vi "MT Decimate Oversampled Waveform.vi"(0 "input complex waveform":T1={"t0"=0.0, "dt"=1.0, "Y"=[]} {"Y" format="%.3f"; "dt" format="%^.2e"; "t0" format="%.4f"}, 5 "decimation factor":i32=16, 7 "offset":i32, 11 "error in (no error)":errorcluster, 13 "reset? (T)":bool=TRUE) -> (4 "output complex waveform":T1 {"Y" format="%.3f"; "dt" format="%^.2e"; "t0" format="%.4f"}, 15 "error out":errorcluster)   [LabVIEW 2020, in "niDMT.lvlib"]
doc: "Decimates the <B>input complex waveform</B> and returns the decimated <B>output complex waveform</B>. Use this VI to decimate the matched filtered waveform at the output of the MT Matched Filter VI to recover the symbols corresponding to the ideal symbol timing location."
uses:
  <vilib>/addons/Modulation/niDMT.lvlib
  <vilib>/addons/Modulation/Analog/controls/Complex Data Waveform.ctl
  <vilib>/addons/Modulation/Analog/support/Validators/mod_Validate Complex Waveform.vi
  <vilib>/addons/Modulation/Analog/support/Validators/mod_WFErrorHandler.vi
  <vilib>/addons/Modulation/niAMT.lvlib
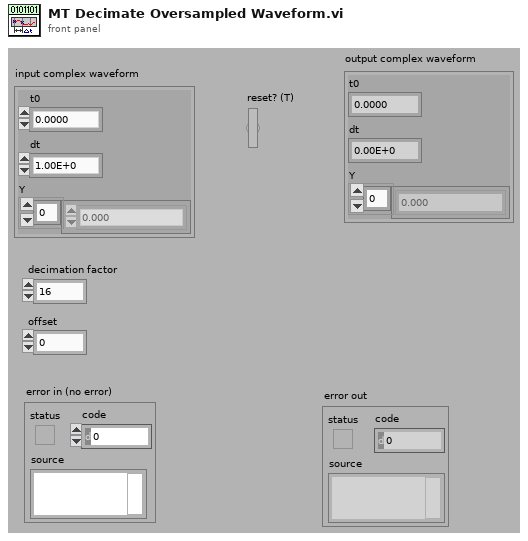
[diagram p1: front panel]
types:
  T1 = typedef "niAMT.lvlib/Complex Data Waveform.ctl" = cluster{"t0":dbl, "dt":dbl, "Y":cdb[]}
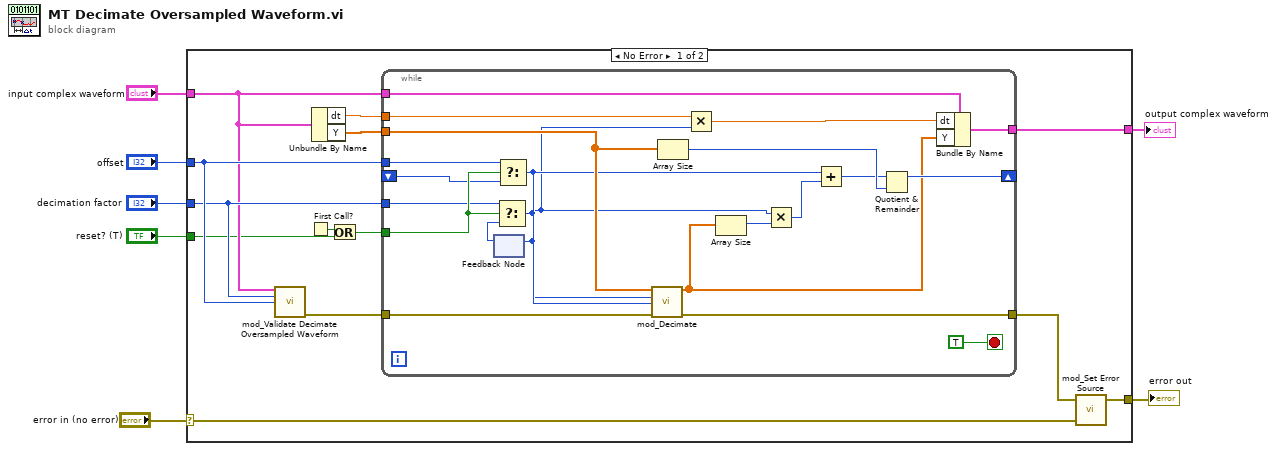
[diagram p0: block diagram]
diagram:
  n1 = case shown="No Error" "error in (no error)" {
    selector: "error in (no error)" -> [w11 w42]
    tunnel: "input complex waveform" -> [w16 _]
    tunnel: "decimation factor" -> [w17 _]
    tunnel: "offset" -> [w19 _]
    tunnel: [w14 _] -> w3
    tunnel: [w13 w42] -> w2
    tunnel: "reset? (T)" -> [w10 _]
    frame No Error {
      n2 = call <vilib>:"mod_Validate Decimate Oversampled Waveform.vi"("input complex waveform"=w16, "decimation factor"=w17, "offset"=w19) -> ("error out"=w15:errorcluster)  [unwired: 12 out]
      n3 = First Call?() -> (First Call?: T/F=w8:bool)
      n4 = Unbundle By Name(w16) -> ("dt"=w18:dbl, "Y"=w20:cdb[])
      n5 = Or(x=w8, y=w10) -> (x .or. y?=w9:bool)
      n6 = while {
        tunnel: w20 -> [w30]
        tunnel: w19 -> [w28]
        tunnel: w18 -> [w41]
        tunnel: w17 -> [w27]
        tunnel: w16 -> [w40]
        tunnel: w15 -> [w35]
        tunnel: [w39] -> w14
        tunnel: [w38] -> w12
        tunnel: w9 -> [w29]
        shift-right: [w33] -> _
        shift-left: _ -> [w23]
        stop <- TRUE stop-if-true
        n7 = feedback #1() -> (w26:i32)  [unwired: 1 out]
        n8 = Select(t=w27, s=w29, f=w26) -> (s? t:f=w21:i32)
        n9 = feedback-in #1(w21) -> ()
        n10 = Select(t=w28, s=w29, f=w23) -> (s? t:f=w22:i32)
        n11 = call <vilib>:"mod_Decimate.vi"("Signal In"=w30, "Samples Per Symbol (16)"=w21, "Offset"=w22, "error in (no error)"=w35) -> ("Signal Out"=w31:cdb[], "error out"=w38:errorcluster)  [unwired: 10 out]
        n12 = Array Size(array=w30) -> (size(s)=w34:i32)
        n13 = Multiply(x=w41, y=w21) -> (x*y=w37:dbl)
        n14 = Array Size(array=w31) -> (size(s)=w25:i32)
        n15 = Multiply(x=w21, y=w25) -> (x*y=w32:i32)
        n16 = Add(x=w22, y=w32) -> (x+y=w24:i32)
        n17 = Quotient & Remainder(x=w24, y=w34) -> (x-y*floor(x/y)=w33:i32)  [unwired: 1 out]
        n18 = Bundle By Name(cluster=w40, "dt"=w37, "Y"=w31) -> (w39:T1)
      }
      n19 = call <vilib>:"mod_Set Error Source.vi"("initial error in (no error)"=w11, "final error in (no error)"=w12) -> ("error out"=w13:errorcluster)  [unwired: 3 out]
    }
    frame Error {
    }
  }
  "output complex waveform" <- w3
  "error out" <- w2
